vi "auto_alignment-v3-2.vi"(0 "pd-plt":refnum<vi>, 1 "xStart":dbl=264.0 format="%#_13g", 2 "yStart":dbl=123.0 format="%#_13g", 3 "NM-params":T2={"alpha"=1.0, "gamma"=2.0, "rho"=0.5, "sigma"=0.5, "simplex L"=0.5}, 5 "alignmnet points":dbl=20.0 format="%#_13g", 7 "stage-refs":T1, 8 "nPts":refnum<vi>, 9 "meter-error":errorcluster, 11 "stage-error":errorcluster, 12 "bar-note":u8, 13 "meas#":dbl format="%#_13g") -> (4 "Optimized Location":dbl[](array[numeric]), 6 "logfile-line-out":string, 10 "meter-error-out":errorcluster, 14 "run time (s)":dbl, 15 "stage-error-out":errorcluster)   [LabVIEW 2024]
uses:
  C:/Users/hpDIRC/Desktop/eic_dirc_daq-LabVIEW_new/Thorlabs/Thorlabs.MotionControl.IntegratedStepperMotorsCLI.dll
  Thorlabs/Thorlabs.MotionControl.IntegratedStepperMotorsCLI.dll
  C:/Users/hpDIRC/Desktop/eic_dirc_daq-LabVIEW_new/Thorlabs/Thorlabs.MotionControl.Benchtop.StepperMotorCLI.dll
  Thorlabs/Thorlabs.MotionControl.Benchtop.StepperMotorCLI.dll
  5b59031f-b1ff-41af-80a7-e72a33ebffa1.vi
  <vilib>/Analysis/baseanly.llb/Real Dot Product.vi
  <vilib>/Array/Sort 2D Array - Pop Stack.vi
  <vilib>/Array/Sort 2D Array - Push Stack.vi
  5b59031f-b1ff-41af-80a7-e72a33ebffa1.vi/269d4b3b-47f5-49e3-8884-44851e4dd9d5.vi
  5b59031f-b1ff-41af-80a7-e72a33ebffa1.vi/6d99389c-673d-4efb-bf33-19b32bcf4cf8.vi
  <vilib>/Analysis/NI_AALBase.lvlib
  <vilib>/Analysis/NI_AALPro.lvlib
panel:
  in  "meter-visa":refnum<visa-resource-name>
  out "z-angle converge":bool
  in  "z-angle-limit":dbl=0.04 caption="Z-Angle Convergence Goal"
  in  "squError-limit":dbl=0.04 caption="Squared Error Convergence Goal"
  out "angle-to-z":dbl
  out "squared error limit":bool
  out "SquError":dbl
  out "x_c":dbl[](array[numeric])
  out "x_e":dbl[](array[numeric])
  out "x_r":dbl[](array[numeric])
  out "x_o":dbl[](array[numeric])
  out "termination-test-simplex":dbl[][](array[numeric])
  out "timeout":bool
  out "simplex converge":bool
  out "value converge":bool
  out "simplex leg lengths":dbl[](array[numeric])
  out "std dev of simplex values":dbl
  out "nPts tested":dbl
  in  "simplex-limit":dbl=1e-06 caption="Simplex Length Convergence Goal" format="%#_13g"
  in  "value-limit":dbl=1e-06 caption="Value Convergence Goal" format="%#_13g"
  out "Pts Tested":dbl[][](array[numeric])
  in  "stop":bool
  # "Test Sub-Points"
  # "centroid"
  # "reflection point"
  # "expansion point"
  # "contraction point"
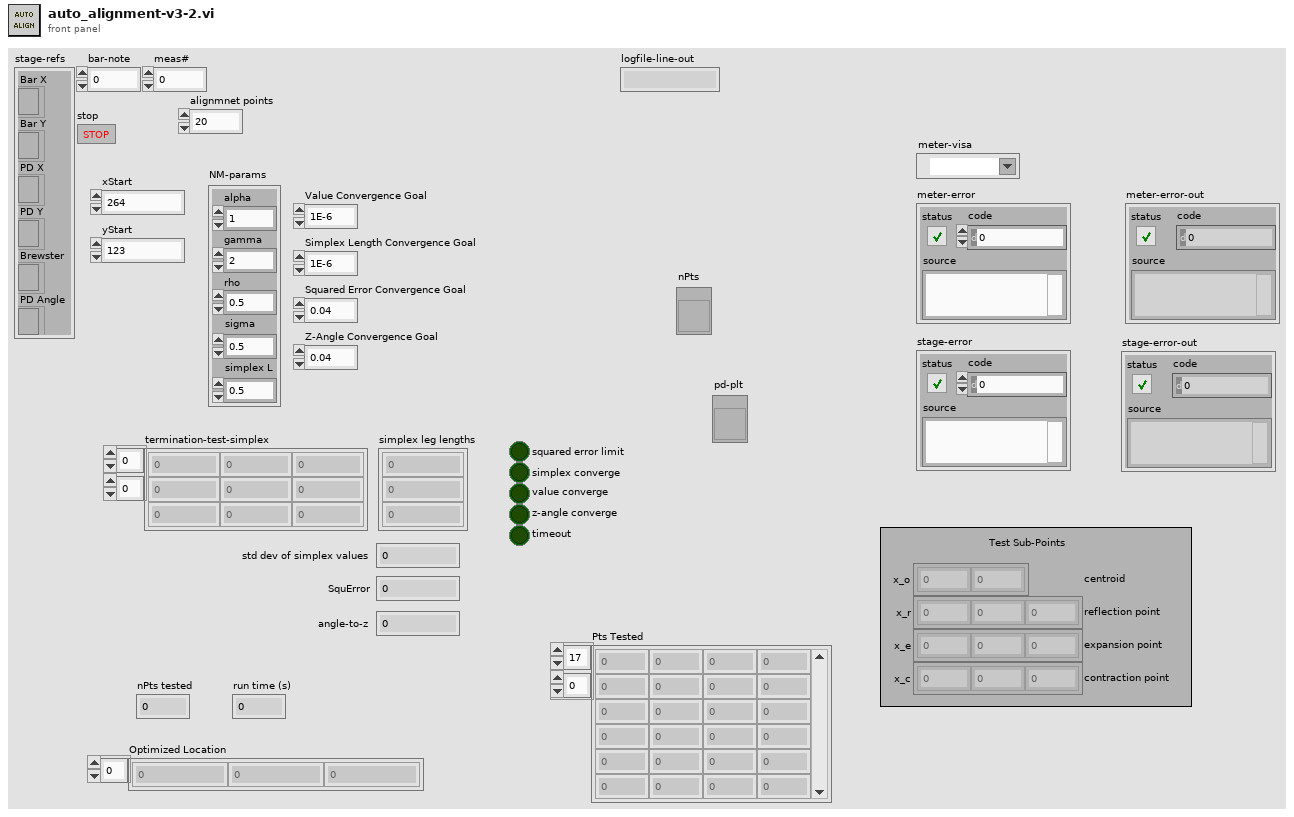
[diagram p1: front panel]
types:
  T1 = cluster{"Bar X":refnum<k24>, "Bar Y":refnum<k24>, "PD X":refnum<k24>, "PD Y":refnum<k24>, "Brewster":refnum<k24>, "PD Angle":refnum<k24>}
  T2 = cluster{"alpha":dbl, "gamma":dbl, "rho":dbl, "sigma":dbl, "simplex L":dbl}
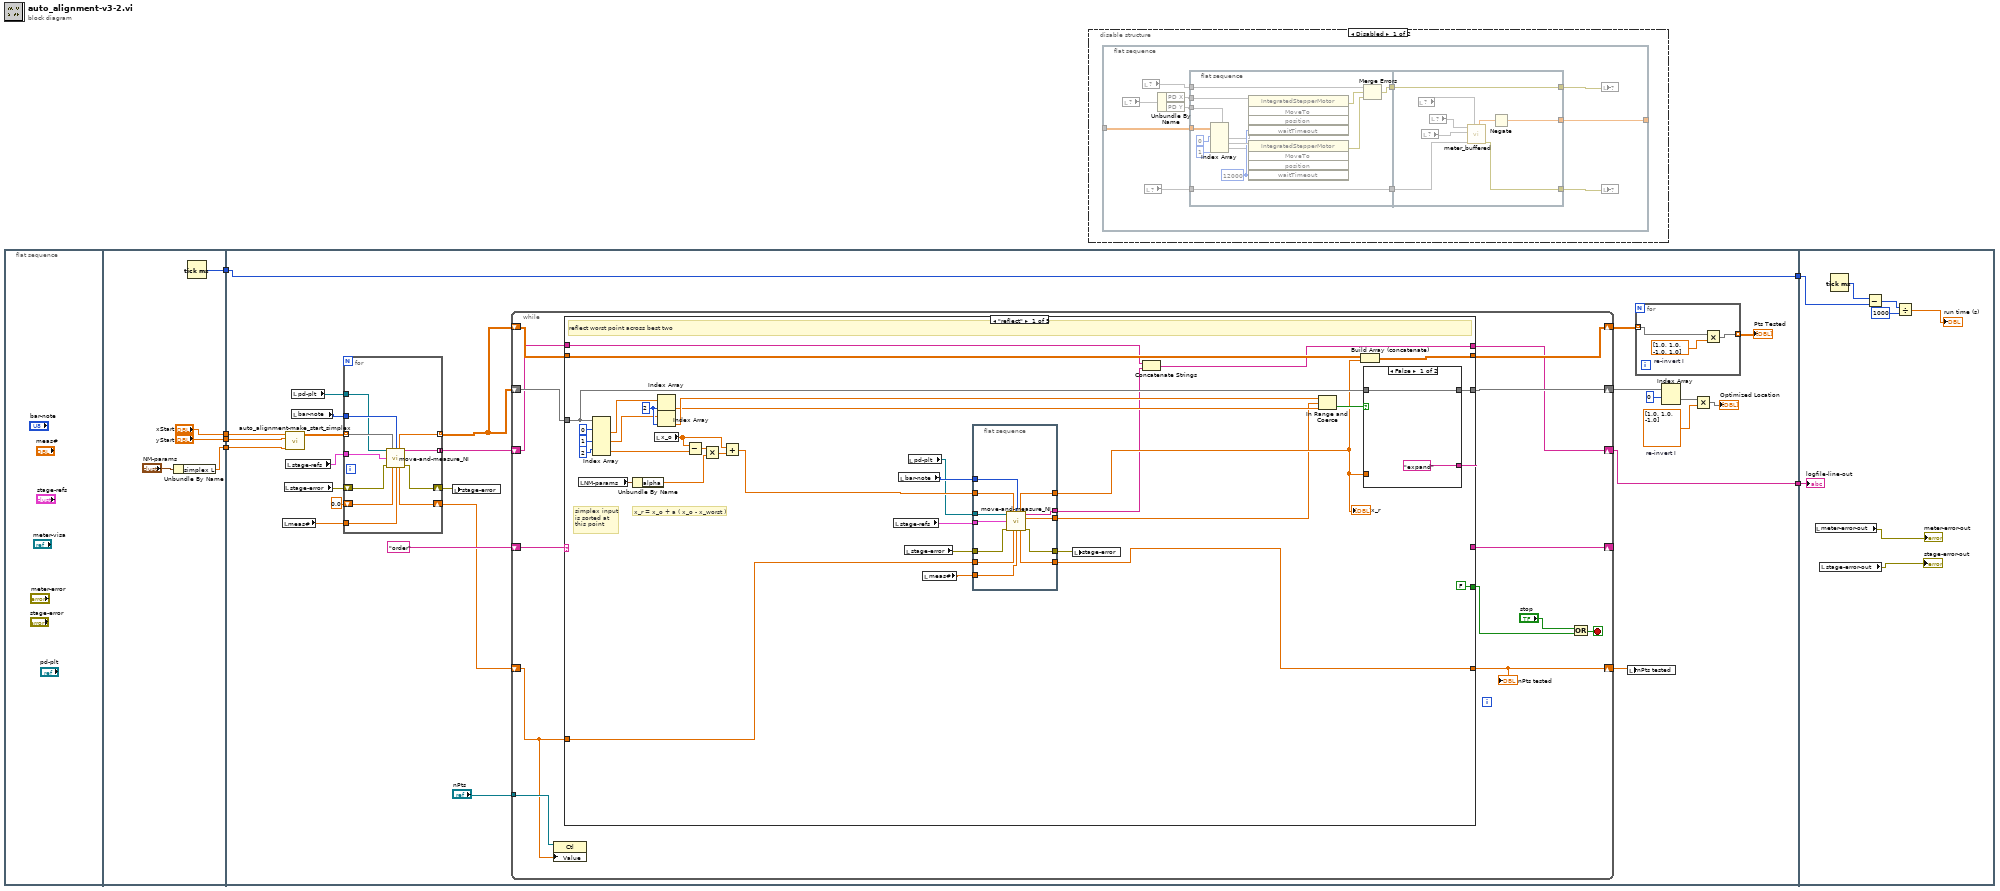
[diagram p0: block diagram]
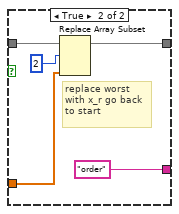
[diagram p3: hidden frame]
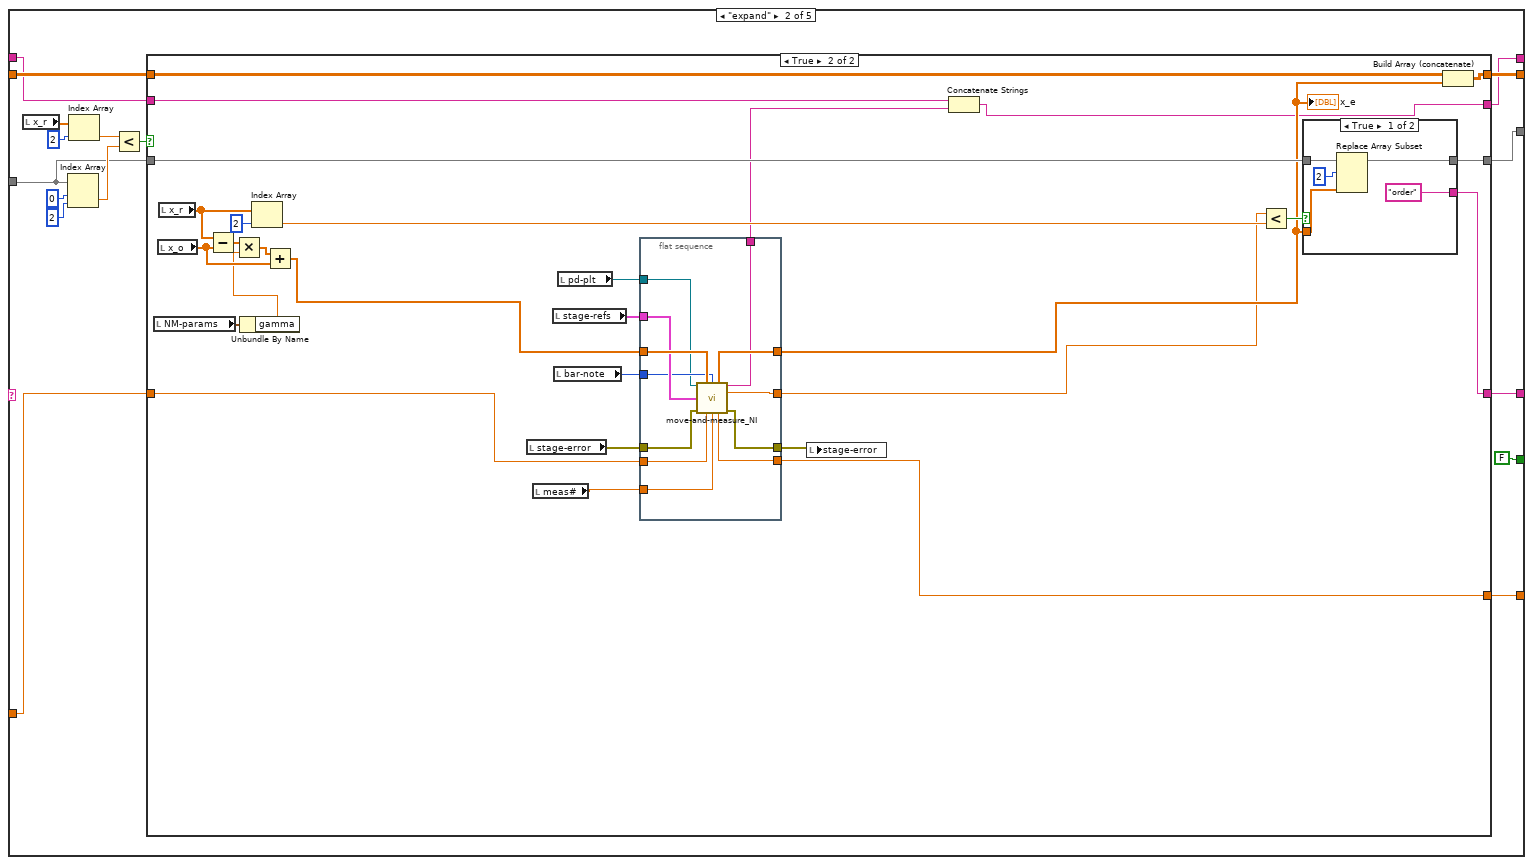
[diagram p4: hidden frame]
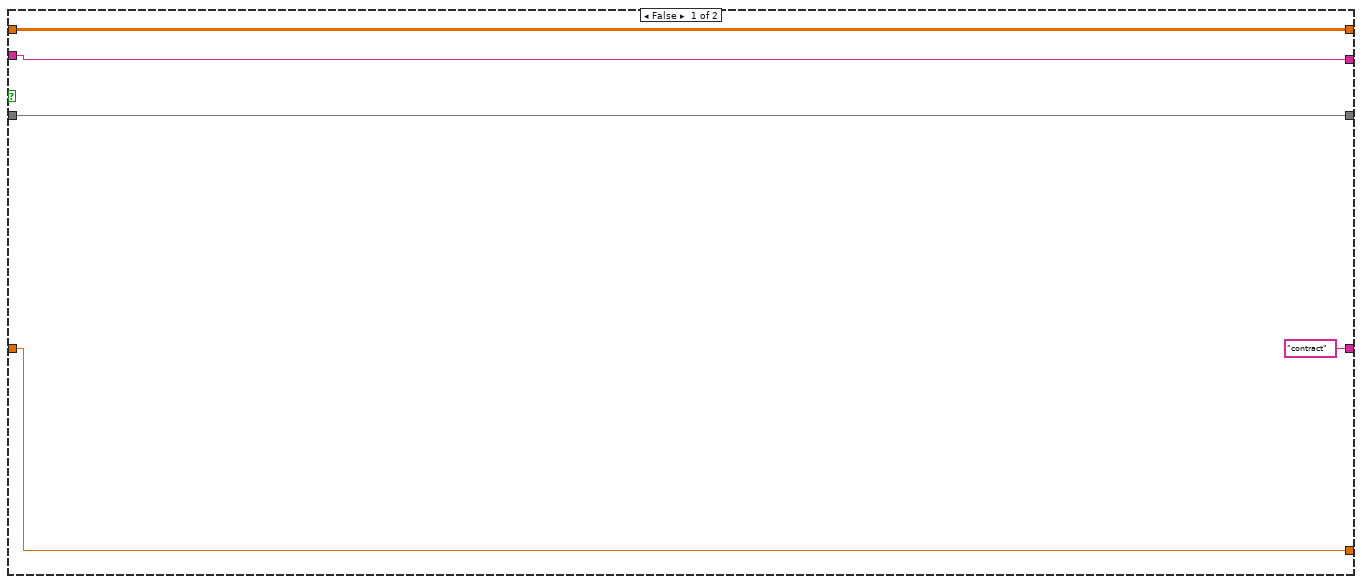
[diagram p5: hidden frame]
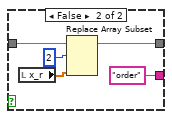
[diagram p6: hidden frame]
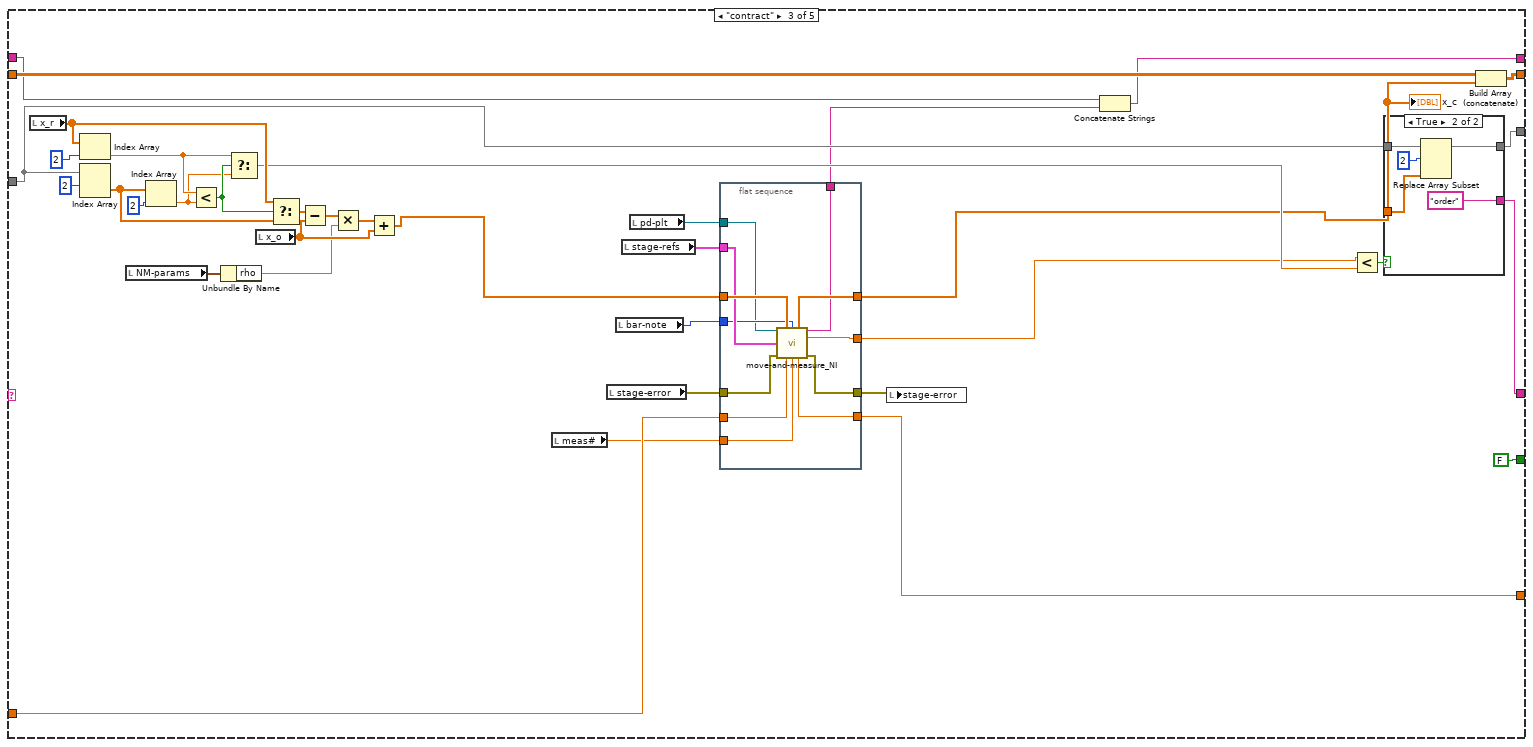
[diagram p7: hidden frame]
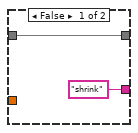
[diagram p8: hidden frame]
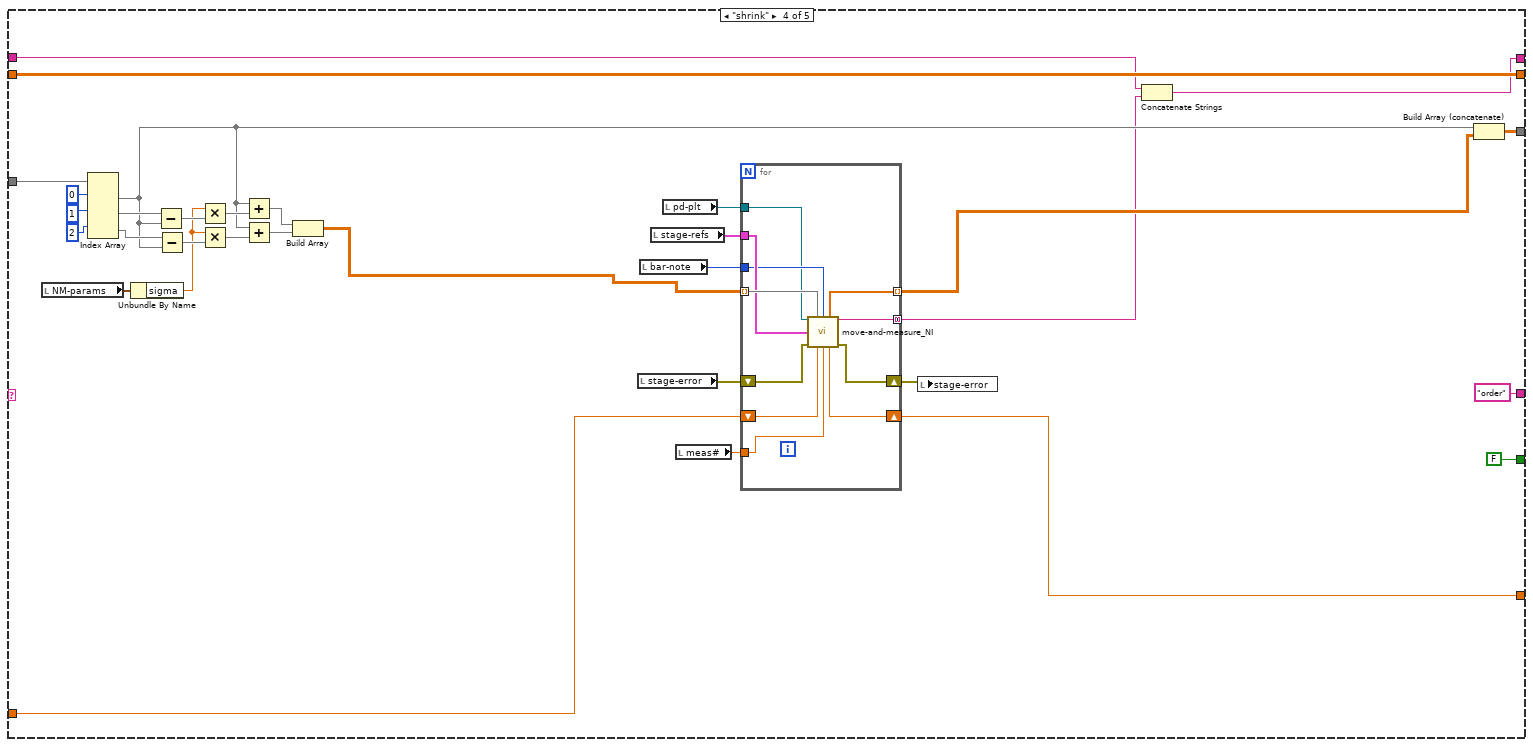
[diagram p9: hidden frame]
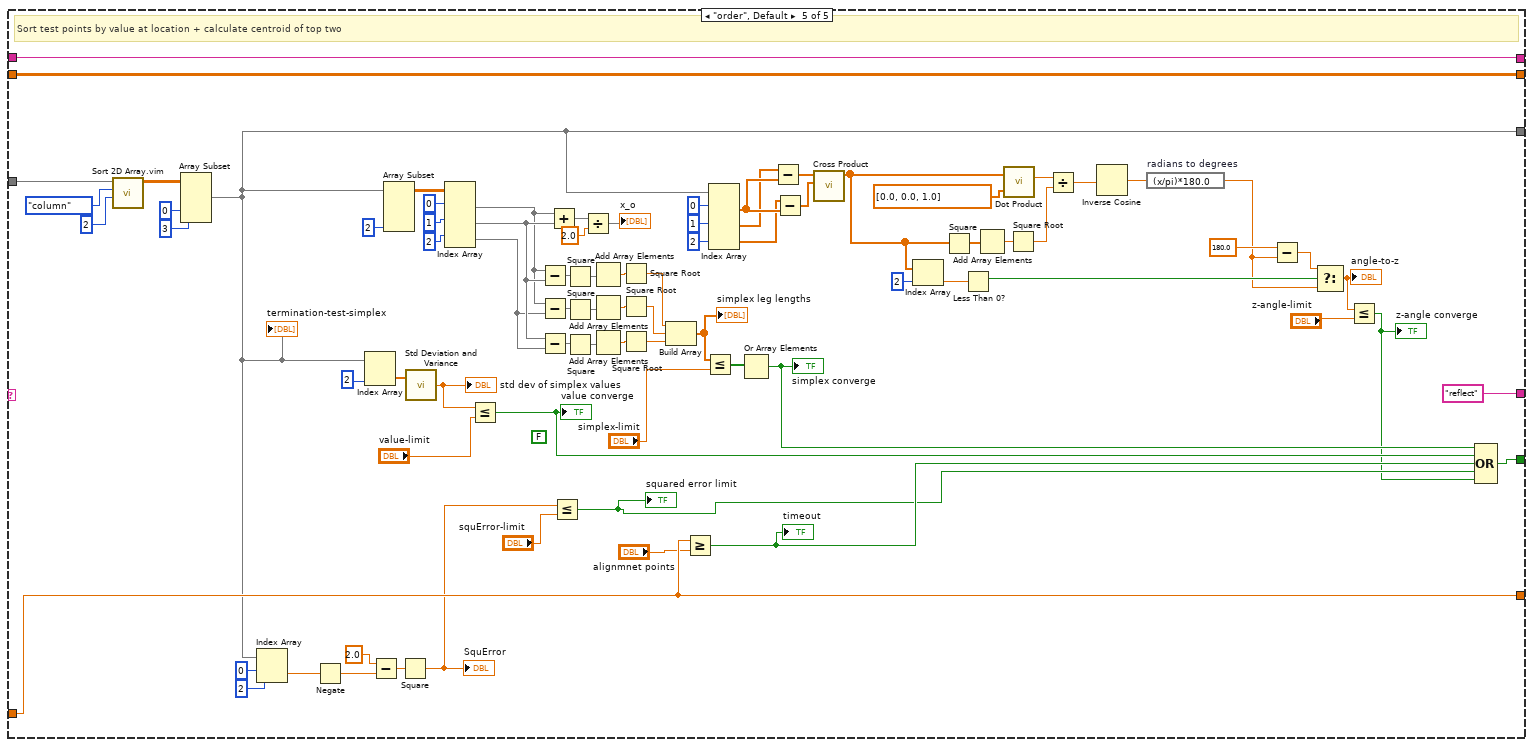
[diagram p10: hidden frame]
diagram:
  n1 = flat-sequence {
    tunnel: [w11] -> w6
    tunnel: ["yStart"] -> w4
    tunnel: ["xStart"] -> w3
    tunnel: [w9] -> w2
    tunnel: w6 -> [w36]
    tunnel: [w36] -> w5
    tunnel: w4 -> [w27]
    tunnel: w3 -> [w28]
    tunnel: w2 -> [w26]
    tunnel: [w17] -> w1
    tunnel: w5 -> [w376]
    tunnel: w1 -> [w370]
    frame #0 {
    }
    frame #1 {
      n2 = Unbundle By Name("NM-params") -> ("simplex L"=w9:dbl)
      n3 = Tick Count (ms)() -> (millisecond timer value=w11:u32)
    }
    frame #2 {
      w31 = dbl[] [1.0, 1.0, -1.0]  # re-invert I
      n4 = local read "meas#"() -> (w15:dbl)
      n5 = local read "stage-error"() -> (w20:errorcluster)
      n6 = call "auto_alignment-make_start_simplex.vi"("L"=w26, "yStart"=w27, "xStart"=w28) -> ("Array"=w29:dbl[][])  [unwired: 8 in]
      n7 = local read "stage-refs"() -> (w13:T1)
      n8 = local read "pd-plt"() -> (w12:refnum<vi>)
      n9 = local read "bar-note"() -> (w16:u8)
      n10 = for {
        shift-right: [w46] -> w24
        shift-left: 0.0 -> [w47]
        tunnel: w29 -> [w51] mode=indexing
        tunnel: [w50] -> w25 mode=indexing
        shift-right: [w48] -> w19
        shift-left: w20 -> [w49]
        tunnel: [w45] -> w18 mode=concatenating
        tunnel: w16 -> [w44]
        tunnel: w15 -> [w43]
        tunnel: w13 -> [w42]
        tunnel: w12 -> [w41]
        n11 = call "move-and-measure_NI.vi"("PD_plots"=w41, "XY-in"=w51, "bar-note"=w44, "stage-refs"=w42, "stage-error-in"=w49, "counter-in"=w47, "meas#"=w43) -> ("measured-point out"=w50:dbl[], "logfile-line-out"=w45:string, "counter-out"=w46:dbl, "stage-error-out"=w48:errorcluster)  [unwired: 4 in, 1 out]
      }
      n12 = local write "stage-error"(w19) -> ()
      n13 = while {
        shift-right: [w63] -> w35
        shift-left: w25 -> [w62]
        shift-right: [w64] -> _
        shift-left: "order" -> [w65]
        shift-right: [w60] -> w22
        shift-left: w25 -> [w61]
        shift-right: [w56] -> w23
        shift-left: w24 -> [w52]
        shift-right: [w54] -> w17
        shift-left: w18 -> [w55]
        tunnel: "nPts" -> [w53]
        stop <- w57 stop-if-true
        n14 = property class="Ctl"(reference=w53, "Value"=w52) -> ()  [unwired: 1 in, 2 out]
        n15 = case shown="\"reflect\"" w65 {
          tunnel: w62 -> [w86 w129 w214 w277 w335]
          tunnel: [FALSE FALSE FALSE FALSE w342] -> w59
          tunnel: [w85 w128 w215 w266 w313] -> w63
          tunnel: [w87 w127 w216 "order" "reflect"] -> w64
          tunnel: w61 -> [w83 w125 w210 w264 w339]
          tunnel: [w82 w124 w209 w264 w339] -> w60
          tunnel: w52 -> [w77 w123 w199 w257 w333]
          tunnel: [w76 w122 w200 w256 w333] -> w56
          tunnel: w55 -> [w72 w120 w195 w251 w290]
          tunnel: [w71 w121 w197 w252 w290] -> w54
          frame "reflect" {
            w94 = 2 ("index")
            # "simplex input\nis sorted at\nthis point"
            # "x_r = x_o + a ( x_o - x_worst )"
            # "reflect worst point across best two"
            n16 = local read "NM-params"() -> (w81:T2)
            n17 = Index Array(array=w86, index (row) #1=0 ("index (row)"), index (row) #2=1 ("index (row)"), index (row) #3=2 ("index (row)")) -> (element #1=w93:dbl[], element #2=w92:dbl[], element #3=w95:dbl[])  [unwired: 3 in]
            n18 = Unbundle By Name(w81) -> ("alpha"=w80:dbl)
            n19 = local read "x_o"() -> (w88:dbl[])
            n20 = Index Array(array=w93, index=w94) -> (element=w90:dbl)
            n21 = Index Array(array=w92, index=w94) -> (element=w91:dbl)
            n22 = Subtract(x=w88, y=w95) -> (x-y=w99:dbl[])
            n23 = Multiply(x=w99, y=w80) -> (x*y=w98:dbl[])
            n24 = Add(x=w88, y=w98) -> (x+y=w74:dbl[])
            n25 = local read "stage-refs"() -> (w67:T1)
            n26 = local read "bar-note"() -> (w69:u8)
            n27 = local read "stage-error"() -> (w79:errorcluster)
            n28 = local read "pd-plt"() -> (w66:refnum<vi>)
            n29 = local read "meas#"() -> (w68:dbl)
            n30 = flat-sequence {
              tunnel: [w112] -> w78
              tunnel: w79 -> [w111]
              tunnel: w77 -> [w110]
              tunnel: w74 -> [w109]
              tunnel: [w108] -> w75
              tunnel: [w107] -> w76
              tunnel: [w103] -> w73
              tunnel: [w106] -> w70
              tunnel: w69 -> [w105]
              tunnel: w68 -> [w104]
              tunnel: w67 -> [w102]
              tunnel: w66 -> [w101]
              frame #0 {
                n31 = call "move-and-measure_NI.vi"("PD_plots"=w101, "XY-in"=w109, "bar-note"=w105, "stage-refs"=w102, "stage-error-in"=w111, "counter-in"=w110, "meas#"=w104) -> ("measured-point out"=w108:dbl[], "logfile-line-out"=w106:string, "iCorr-out"=w103:dbl, "counter-out"=w107:dbl, "stage-error-out"=w112:errorcluster)  [unwired: 4 in]
              }
            }
            n32 = local write "stage-error"(w78) -> ()
            n33 = Concatenate Strings(w72, w70) -> (w71:string)
            n34 = In Range and Coerce(upper limit=w91, x=w73, lower limit=w90) -> (In Range?=w89:bool)  [unwired: 1 out]
            n35 = Build Array (concatenate)(w83, w75) -> (w82:dbl[][])
            n36 = case shown="False" w89 {
              tunnel: ["expand" "order"] -> w87
              tunnel: w86 -> [w113 w119]
              tunnel: [w113 w116] -> w85
              tunnel: w75 -> [_ w117]
              frame False {
              }
              frame True {
                # "replace worst \nwith x_r go back\nto start"
                n37 = Replace Array Subset(array=w119, new element=w117, index (row)=2) -> (w116:dbl[][])  [unwired: 1 in]
              }
            }
            "x_r" <- w75
          }
          frame "expand" {
            n38 = local read "x_r"() -> (w134:dbl[])
            n39 = Index Array(array=w129, index (row)=0, index (col)=2 ("disabled index (col)")) -> (element=w132:dbl)
            n40 = Index Array(array=w134, index=2) -> (element=w131:dbl)
            n41 = Less?(x=w131, y=w132) -> (x < y?=w130:bool)
            n42 = case shown="True" w130 {
              tunnel: w129 -> [w141 w162]
              tunnel: [w141 w161] -> w128
              tunnel: ["contract" w160] -> w127
              tunnel: w125 -> [w139 w159]
              tunnel: [w139 w158] -> w124
              tunnel: w123 -> [w138 w151]
              tunnel: [w138 w150] -> w122
              tunnel: [w137 w147] -> w121
              tunnel: w120 -> [w137 w145]
              frame False {
              }
              frame True {
                n43 = local read "NM-params"() -> (w157:T2)
                n44 = local read "x_o"() -> (w167:dbl[])
                n45 = local read "x_r"() -> (w166:dbl[])
                n46 = Subtract(x=w166, y=w167) -> (x-y=w169:dbl[])
                n47 = Unbundle By Name(w157) -> ("gamma"=w156:dbl)
                n48 = Multiply(x=w169, y=w156) -> (x*y=w168:dbl[])
                n49 = Index Array(array=w166, index=2) -> (element=w164:dbl)
                n50 = Add(x=w168, y=w167) -> (x+y=w153:dbl[])
                n51 = local read "stage-error"() -> (w155:errorcluster)
                n52 = local read "meas#"() -> (w143:dbl)
                n53 = local read "stage-refs"() -> (w148:T1)
                n54 = local read "bar-note"() -> (w144:u8)
                n55 = local read "pd-plt"() -> (w142:refnum<vi>)
                n56 = flat-sequence {
                  tunnel: [w181] -> w154
                  tunnel: w155 -> [w180]
                  tunnel: w151 -> [w179]
                  tunnel: w153 -> [w178]
                  tunnel: [w177] -> w152
                  tunnel: [w176] -> w150
                  tunnel: [w175] -> w149
                  tunnel: w148 -> [w174]
                  tunnel: [w173] -> w146
                  tunnel: w144 -> [w172]
                  tunnel: w143 -> [w171]
                  tunnel: w142 -> [w170]
                  frame #0 {
                    n57 = call "move-and-measure_NI.vi"("PD_plots"=w170, "XY-in"=w178, "bar-note"=w172, "stage-refs"=w174, "stage-error-in"=w180, "counter-in"=w179, "meas#"=w171) -> ("measured-point out"=w177:dbl[], "logfile-line-out"=w173:string, "iCorr-out"=w175:dbl, "counter-out"=w176:dbl, "stage-error-out"=w181:errorcluster)  [unwired: 4 in]
                  }
                }
                n58 = local write "stage-error"(w154) -> ()
                n59 = Concatenate Strings(w145, w146) -> (w147:string)
                n60 = Less?(x=w149, y=w164) -> (x < y?=w163:bool)
                n61 = case shown="True" w163 {
                  tunnel: w162 -> [w185 w190]
                  tunnel: w152 -> [w184 _]
                  tunnel: [w183 w189] -> w161
                  tunnel: ["order" "order"] -> w160
                  frame True {
                    n62 = Replace Array Subset(array=w185, new element=w184, index (row)=2) -> (w183:dbl[][])  [unwired: 1 in]
                  }
                  frame False {
                    n63 = local read "x_r"() -> (w187:dbl[])
                    n64 = Replace Array Subset(array=w190, new element=w187, index (row)=2) -> (w189:dbl[][])  [unwired: 1 in]
                  }
                }
                n65 = Build Array (concatenate)(w159, w152) -> (w158:dbl[][])
                "x_e" <- w152
              }
            }
          }
          frame "contract" {
            n66 = local read "x_r"() -> (w224:dbl[])
            n67 = Index Array(array=w224, index=2) -> (element=w219:dbl)
            n68 = Index Array(array=w214, index (row)=2) -> (element=w223:dbl[])  [unwired: 1 in]
            n69 = local read "NM-params"() -> (w208:T2)
            n70 = Index Array(array=w223, index=2) -> (element=w218:dbl)
            n71 = Less?(x=w219, y=w218) -> (x < y?=w220:bool)
            n72 = Unbundle By Name(w208) -> ("rho"=w207:dbl)
            n73 = Select(t=w219, s=w220, f=w218) -> (s? t:f=w206:dbl)
            n74 = local read "x_o"() -> (w212:dbl[])
            n75 = Select(t=w224, s=w220, f=w223) -> (s? t:f=w222:dbl[])
            n76 = Subtract(x=w222, y=w212) -> (x-y=w221:dbl[])
            n77 = Multiply(x=w221, y=w207) -> (x*y=w213:dbl[])
            n78 = Add(x=w213, y=w212) -> (x+y=w203:dbl[])
            n79 = local read "meas#"() -> (w193:dbl)
            n80 = local read "stage-error"() -> (w205:errorcluster)
            n81 = local read "bar-note"() -> (w194:u8)
            n82 = local read "stage-refs"() -> (w198:T1)
            n83 = local read "pd-plt"() -> (w192:refnum<vi>)
            n84 = flat-sequence {
              tunnel: [w239] -> w204
              tunnel: w205 -> [w238]
              tunnel: w199 -> [w237]
              tunnel: w203 -> [w236]
              tunnel: [w235] -> w202
              tunnel: [w234] -> w200
              tunnel: [w233] -> w201
              tunnel: w198 -> [w232]
              tunnel: [w231] -> w196
              tunnel: w194 -> [w230]
              tunnel: w193 -> [w229]
              tunnel: w192 -> [w228]
              frame #0 {
                n85 = call "move-and-measure_NI.vi"("PD_plots"=w228, "XY-in"=w236, "bar-note"=w230, "stage-refs"=w232, "stage-error-in"=w238, "counter-in"=w237, "meas#"=w229) -> ("measured-point out"=w235:dbl[], "logfile-line-out"=w231:string, "iCorr-out"=w233:dbl, "counter-out"=w234:dbl, "stage-error-out"=w239:errorcluster)  [unwired: 4 in]
              }
            }
            n86 = local write "stage-error"(w204) -> ()
            n87 = Concatenate Strings(w195, w196) -> (w197:string)
            n88 = Less?(x=w201, y=w206) -> (x < y?=w217:bool)
            n89 = case shown="True" w217 {
              tunnel: ["shrink" "order"] -> w216
              tunnel: [w240 w242] -> w215
              tunnel: w214 -> [w240 w244]
              tunnel: w202 -> [_ w243]
              frame False {
              }
              frame True {
                n90 = Replace Array Subset(array=w244, new element=w243, index (row)=2) -> (w242:dbl[][])  [unwired: 1 in]
              }
            }
            n91 = Build Array (concatenate)(w210, w202) -> (w209:dbl[][])
            "x_c" <- w202
          }
          frame "shrink" {
            n92 = local read "NM-params"() -> (w261:T2)
            n93 = Index Array(array=w277, index (row) #1=0 ("index (row)"), index (row) #2=1 ("index (row)"), index (row) #3=2 ("index (row)")) -> (element #1=w267:dbl[], element #2=w273:dbl[], element #3=w272:dbl[])  [unwired: 3 in]
            n94 = Unbundle By Name(w261) -> ("sigma"=w260:dbl)
            n95 = Subtract(x=w273, y=w267) -> (x-y=w270:dbl[])
            n96 = Subtract(x=w272, y=w267) -> (x-y=w271:dbl[])
            n97 = Multiply(x=w260, y=w270) -> (x*y=w269:dbl[])
            n98 = Multiply(x=w260, y=w271) -> (x*y=w268:dbl[])
            n99 = Add(x=w267, y=w269) -> (x+y=w263:dbl[])
            n100 = Add(x=w267, y=w268) -> (x+y=w262:dbl[])
            n101 = Build Array(w263, w262) -> (w254:dbl[][])
            n102 = local read "stage-error"() -> (w258:errorcluster)
            n103 = local read "bar-note"() -> (w249:u8)
            n104 = local read "stage-refs"() -> (w253:T1)
            n105 = local read "pd-plt"() -> (w247:refnum<vi>)
            n106 = local read "meas#"() -> (w248:dbl)
            n107 = for {
              shift-right: [w286] -> w256
              shift-left: w257 -> [w287]
              tunnel: w254 -> [w289] mode=indexing
              tunnel: [w288] -> w255 mode=indexing
              shift-right: [w284] -> w259
              shift-left: w258 -> [w285]
              tunnel: w253 -> [w283]
              tunnel: [w282] -> w250 mode=concatenating
              tunnel: w249 -> [w281]
              tunnel: w248 -> [w280]
              tunnel: w247 -> [w279]
              n108 = call "move-and-measure_NI.vi"("PD_plots"=w279, "XY-in"=w289, "bar-note"=w281, "stage-refs"=w283, "stage-error-in"=w285, "counter-in"=w287, "meas#"=w280) -> ("measured-point out"=w288:dbl[], "logfile-line-out"=w282:string, "counter-out"=w286:dbl, "stage-error-out"=w284:errorcluster)  [unwired: 4 in, 1 out]
            }
            n109 = local write "stage-error"(w259) -> ()
            n110 = Concatenate Strings(w251, w250) -> (w252:string)
            n111 = Build Array (concatenate)(w267, w255) -> (w266:dbl[][])
          }
          frame "order", Default {
            (unwired) FALSE
            # "Sort test points by value at location + calculate centroid of top two"
            n112 = call "Sort 2D Array.vim"("index"=2, "dimension to index (column)"=enum16{"column", "row"}."column", "2D array"=w335) -> ("sorted 2D array"=w334:dbl[][])  [unwired: 7 in, 1 out]
            n113 = Array Subset(array=w334, index (col)=0 ("index"), length (col)=3 ("length")) -> (w313:dbl[][])  [unwired: 2 in]
            "termination-test-simplex" <- w313
            n114 = Index Array(array=w313, index (row)=0, index (col)=2 ("disabled index (col)")) -> (element=w328:dbl)
            n115 = Negate(x=w328) -> (-x=w326:dbl)
            n116 = Index Array(array=w313, index (col)=2 ("index")) -> (element=w359:dbl[])  [unwired: 1 in]
            n117 = Subtract(x=2.0, y=w326) -> (x-y=w327:dbl)
            n118 = Array Subset(array=w313, length (col)=2 ("length")) -> (w358:dbl[][])  [unwired: 3 in]
            n119 = Square(x=w327) -> (x^2=w325:dbl)
            "SquError" <- w325
            n120 = call <vilib>:"Std Deviation and Variance.vi"("X"=w359) -> ("standard deviation"=w340:dbl)  [unwired: 1 in, 2 out]
            "std dev of simplex values" <- w340
            n121 = Index Array(array=w358, index (row) #1=0 ("index (row)"), index (row) #2=1 ("index (row)"), index (row) #3=2 ("index (row)")) -> (element #1=w323:dbl[], element #2=w324:dbl[], element #3=w322:dbl[])  [unwired: 3 in]
            n122 = Less Or Equal?(x=w340, y="value-limit") -> (x <= y?=w297:bool)
            "value converge" <- w297
            n123 = Subtract(x=w323, y=w324) -> (x-y=w356:dbl[])
            n124 = Subtract(x=w323, y=w322) -> (x-y=w348:dbl[])
            n125 = Subtract(x=w324, y=w322) -> (x-y=w351:dbl[])
            n126 = Add(x=w323, y=w324) -> (x+y=w363:dbl[])
            n127 = Less Or Equal?(x=w325, y="squError-limit") -> (x <= y?=w292:bool)
            "squared error limit" <- w292
            n128 = Square(x=w356) -> (x^2=w355:dbl[])
            n129 = Square(x=w348) -> (x^2=w352:dbl[])
            n130 = Square(x=w351) -> (x^2=w350:dbl[])
            n131 = Divide(x=w363, y=2.0) -> (x/y=→"x_o":dbl[])
            n132 = Add Array Elements(numeric array=w355) -> (sum=w354:dbl)
            n133 = Add Array Elements(numeric array=w352) -> (sum=w353:dbl)
            n134 = Add Array Elements(numeric array=w350) -> (sum=w349:dbl)
            n135 = Square Root(x=w354) -> (sqrt(x)=w345:dbl)
            n136 = Square Root(x=w353) -> (sqrt(x)=w346:dbl)
            n137 = Square Root(x=w349) -> (sqrt(x)=w347:dbl)
            n138 = Build Array(w345, w346, w347) -> (w344:dbl[])
            "simplex leg lengths" <- w344
            n139 = Greater Or Equal?(x=w333, y="alignmnet points") -> (x >= y?=w331:bool)
            "timeout" <- w331
            n140 = Less Or Equal?(x=w344, y="simplex-limit") -> (x <= y?=w343:bool[])
            n141 = Index Array(array=w313, index (row) #1=0 ("index (row)"), index (row) #2=1 ("index (row)"), index (row) #3=2 ("index (row)")) -> (element #1=w309:dbl[], element #2=w308:dbl[], element #3=w307:dbl[])  [unwired: 3 in]
            n142 = Or Array Elements(Boolean array=w343) -> (logical OR=w341:bool)
            "simplex converge" <- w341
            n143 = Subtract(x=w308, y=w309) -> (x-y=w321:dbl[])
            n144 = Subtract(x=w307, y=w309) -> (x-y=w320:dbl[])
            n145 = call <vilib>:"Cross Product.vi"("B Vector"=w320, "A Vector"=w321) -> ("Cross Product"=w305:dbl[])  [unwired: 8 in, 1 out]
            n146 = Index Array(array=w305, index=2) -> (element=w303:dbl)
            n147 = Square(x=w305) -> (x^2=w319:dbl[])
            n148 = Less Than 0?(x=w303) -> (x < 0?=w302:bool)
            n149 = Add Array Elements(numeric array=w319) -> (sum=w318:dbl)
            n150 = call-poly <vilib>:"Dot Product.vi"("Y Vector"=dbl[] [0.0, 0.0, 1.0], "X Vector"=w305) -> ("X * Y"=w316:dbl)  [unwired: 1 out]
            n151 = Square Root(x=w318) -> (sqrt(x)=w315:dbl)
            n152 = Divide(x=w316, y=w315) -> (x/y=w306:dbl)
            n153 = Inverse Cosine(1:w306) -> (0:w314:dbl)
            n154 = expression code="(x/pi)*180.0" "radians to degrees"(w314) -> (w299:dbl)
            n155 = Subtract(x=180.0, y=w299) -> (x-y=w301:dbl)
            n156 = Select(t=w301, s=w302, f=w299) -> (s? t:f=w298:dbl)
            "angle-to-z" <- w298
            n157 = Less Or Equal?(x=w298, y="z-angle-limit") -> (x <= y?=w291:bool)
            "z-angle converge" <- w291
            n158 = Compound Arithmetic op=OR(w341, w297, w331, w292, w291) -> (w342:bool)
          }
        }
        "nPts tested" <- w56
        n159 = Compound Arithmetic op=OR("stop", w59) -> (w57:bool)
      }
      n160 = local write "nPts tested"(w23) -> ()
      n161 = for {
        tunnel: [w39] -> w21 mode=indexing
        tunnel: w22 -> [w40] mode=indexing
        w38 = dbl[] [1.0, 1.0, -1.0, 1.0]  # re-invert I
        n162 = Multiply(x=w40, y=w38) -> (x*y=w39:dbl[])
      }
      "Pts Tested" <- w21
      n163 = Index Array(array=w35, index (row)=0) -> (element=w32:dbl[])  [unwired: 1 in]
      n164 = Multiply(x=w32, y=w31) -> (x*y=→"Optimized Location":dbl[])
    }
    frame #3 {
      n165 = local read "meter-error-out"() -> (→"meter-error-out":errorcluster)
      n166 = local read "stage-error-out"() -> (→"stage-error-out":errorcluster)
      n167 = Tick Count (ms)() -> (millisecond timer value=w377:u32)
      n168 = Subtract(x=w377, y=w376) -> (x-y=w375:u32)
      n169 = Divide(x=w375, y=u32 1000) -> (x/y=→"run time (s)":dbl)
      "logfile-line-out" <- w370
    }
  }
  n170 = disable-structure shown="Disabled" {
    frame Disabled {
      n171 = flat-sequence {
        tunnel: [w386] -> _
        tunnel: [w378] -> _
        frame #0 {
          n172 = local read item#-1() -> (w382)
          n173 = local read item#-1() -> (w383)
          n174 = local read item#-1() -> (w381)
          n175 = Unbundle By Name(w382) -> ("PD X"=w388, "PD Y"=w387)
          n176 = flat-sequence {
            tunnel: w388 -> [w399]
            tunnel: w387 -> [w398]
            tunnel: w383 -> [w392]
            tunnel: [w390] -> w378
            tunnel: w381 -> [w389]
            tunnel: [w391] -> w380
            tunnel: [w389] -> w379
            tunnel: [w409] -> w384
            tunnel: [w406] -> w385
            tunnel: [w402] -> w386
            tunnel: w380 -> [w409]
            tunnel: w379 -> [w407]
            frame #0 {
              w397 = 12000 ("waitTimeout")
              n177 = Index Array(array=w390, index (row) #1=0 ("index"), index (row) #2=1 ("index")) -> (element #1=w394, element #2=w393)  [unwired: 2 in]
              n178 = invoke class="IntegratedStepperMotor" method="MoveTo"(reference=w399, "position"=w394, "waitTimeout"=w397) -> (error out=w401:errorcluster)  [unwired: 2 in, 4 out]
              n179 = invoke class="IntegratedStepperMotor" method="MoveTo"(reference=w398, "position"=w393, "waitTimeout"=w397) -> (error out=w400:errorcluster)  [unwired: 2 in, 4 out]
              n180 = Merge Errors(w392, w401, w400) -> (w391:errorcluster)
            }
            frame #1 {
              n181 = local read item#-1() -> (w405)
              n182 = local read item#-1() -> (w403)
              n183 = local read item#-1() -> (w404)
              n184 = call "meter_buffered.vi"("Samples"=w405, "error in"=w407, "PD ranges"=w403, "meter-VISA"=w404) -> ("error out"=w406:errorcluster, "iCorr"=w408:dbl)  [unwired: 3 in, 3 out]
              n185 = Negate(x=w408) -> (-x=w402:dbl)
            }
          }
          n186 = local write item#-1(w384) -> ()
          n187 = local write item#-1(w385) -> ()
        }
      }
    }
    frame Enabled {
    }
  }
